vi "append log entry - low level.vi"(6 "Record to Add (\"\")":string, 7 "Current Log Contents (\"\")":string) -> (2 "Records":i32, 3 "New Log Contents":string)   [LabVIEW 2011]
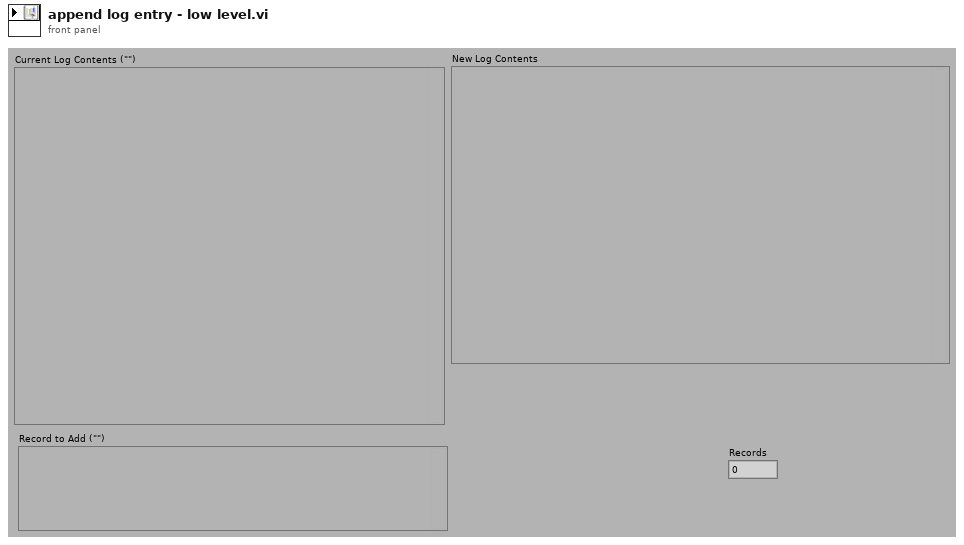
[diagram p1: front panel]
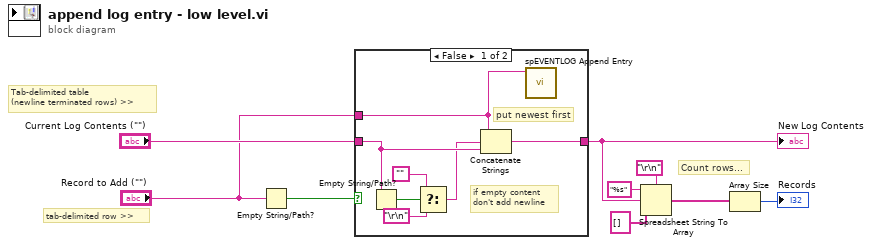
[diagram p0: block diagram]
diagram:
  # "Count rows..."
  # "tab-delimited row >>"
  # "Tab-delimited table\n(newline terminated rows) >>"
  n1 = Empty String/Path?(string/path="Record to Add (\"\")") -> (empty?=w3:bool)
  n2 = case shown="False" w3 {
    tunnel: [w16 w17] -> w8
    tunnel: "Current Log Contents (\"\")" -> [w15 w17]
    tunnel: "Record to Add (\"\")" -> [w10 _]
    frame False {
      # "if empty content\ndon't add newline"
      # "put newest first"
      n3 = Empty String/Path?(string/path=w15) -> (empty?=w14:bool)
      n4 = Select(t="", s=w14, f="\r\n") -> (s? t:f=w12:string)
      n5 = Concatenate Strings(w10, w12, w15) -> (w16:string)
      n6 = call "spEVENTLOG Append Entry.vi"("Log Entry (\"\")"=w10) -> ()  [unwired: 10 in, 1 out]
    }
    frame True {
    }
  }
  "New Log Contents" <- w8
  n7 = Spreadsheet String To Array(delimiter (Tab)="\r\n", format string="%s", spreadsheet string=w8, array type (2D Dbl)=string[] []) -> (array=w5:string[])
  n8 = Array Size(array=w5) -> (size(s)=→"Records":i32)
